vi "HolDrvCtrl_PackControllers.vi"(9 "thetaProfiledPID_CTRL":T1={"Controller"={"Kp"=0.0, "Ki"=0.0, "Kd"=0.0, "Period"=0.0, "Max_Integral"=1.0, "Min_Integral"=-1.0, "Max_Input"=0.0, "Min_Input"=0.0, "Continuous"=FALSE, "PositionError"=0.0, "VelocityError"=0.0, "PrevError"=0.0, "Total_Integral"=0.0, "PositionTolerance"=0.05, "VelocityTolerance"=9.99e+35, "SetPoint"=0.0, "Kf"=0.0, "Prev_Deriv"=0.0, "Prev_Deriv 2"=0.0, "DerivativeFilter"=FALSE, "Min_Output"=-9.99e+35, "Max_Output"=9.9e+35, "Prev_F_P"=0.0, "Prev_F_P_2"=0.0, "AntiWindupActive"=FALSE, "Measurement"=0.0, "IntegralZone"=9.9e+30}, "Goal"={"Position"=0.0, "Velocity"=0.0}, "Setpoint"={"Position"=0.0, "Velocity"=0.0}, "Constraint"={"MaxVelocity"=0.0, "MaxAcceleration"=0.0}} {"Constraint"."MaxAcceleration" format="%16_6e"; "Constraint"."MaxVelocity" format="%16_6e"; "Setpoint"."Velocity" format="%16_6e"; "Setpoint"."Position" format="%16_6e"; "Goal"."Velocity" format="%16_6e"; "Goal"."Position" format="%16_6e"; "Controller"."IntegralZone" format="%16_6e"; "Controller"."Measurement" format="%16_6e"; "Controller"."Prev_F_P_2" format="%16_6e"; "Controller"."Prev_F_P" format="%16_6e"; "Controller"."Max_Output" format="%16_6e"; "Controller"."Min_Output" format="%16_6e"; "Controller"."Prev_Deriv 2" format="%16_6e"; "Controller"."Prev_Deriv" format="%16_6e"; "Controller"."Kf" format="%16_6e"; "Controller"."SetPoint" format="%16_6e"; "Controller"."VelocityTolerance" format="%16_6e"; "Controller"."PositionTolerance" format="%16_6e"; "Controller"."Total_Integral" format="%16_6e"; "Controller"."PrevError" format="%16_6e"; "Controller"."VelocityError" format="%16_6e"; "Controller"."PositionError" format="%16_6e"; "Controller"."Min_Input" format="%16_6e"; "Controller"."Max_Input" format="%16_6e"; "Controller"."Min_Integral" format="%16_6e"; "Controller"."Max_Integral" format="%16_6e"; "Controller"."Period" format="%16_6e"; "Controller"."Kd" format="%16_6e"; "Controller"."Ki" format="%16_6e"; "Controller"."Kp" format="%16_6e"}, 10 "Y PID Tuning":T5={"Kp"=0.0, "Ki"=0.0, "Kd"=0.0, "MaximumIntegral"=9.9e+30, "MinimumIntegral"=-9.9e+30, "IntegralZone"=9.9e+30}, 11 "X PID Tuning":T5={"Kp"=0.0, "Ki"=0.0, "Kd"=0.0, "MaximumIntegral"=9.9e+30, "MinimumIntegral"=-9.9e+30, "IntegralZone"=9.9e+30}) -> (3 "HOLONOMIC_CTRL_PACK_TUNING":T6={"X PID Tuning"={"Kp"=0.0, "Ki"=0.0, "Kd"=0.0, "MaximumIntegral"=9.9e+30, "MinimumIntegral"=-9.9e+30, "IntegralZone"=9.9e+30}, "Y PID Tuning"={"Kp"=0.0, "Ki"=0.0, "Kd"=0.0, "MaximumIntegral"=9.9e+30, "MinimumIntegral"=-9.9e+30, "IntegralZone"=9.9e+30}, "thetaProfiledPID_CTRL"={"Controller"={"Kp"=0.0, "Ki"=0.0, "Kd"=0.0, "Period"=0.0, "Max_Integral"=1.0, "Min_Integral"=-1.0, "Max_Input"=0.0, "Min_Input"=0.0, "Continuous"=FALSE, "PositionError"=0.0, "VelocityError"=0.0, "PrevError"=0.0, "Total_Integral"=0.0, "PositionTolerance"=0.05, "VelocityTolerance"=9.99e+35, "SetPoint"=0.0, "Kf"=0.0, "Prev_Deriv"=0.0, "Prev_Deriv 2"=0.0, "DerivativeFilter"=FALSE, "Min_Output"=-9.99e+35, "Max_Output"=9.9e+35, "Prev_F_P"=0.0, "Prev_F_P_2"=0.0, "AntiWindupActive"=FALSE, "Measurement"=0.0, "IntegralZone"=9.9e+30}, "Goal"={"Position"=0.0, "Velocity"=0.0}, "Setpoint"={"Position"=0.0, "Velocity"=0.0}, "Constraint"={"MaxVelocity"=0.0, "MaxAcceleration"=0.0}}} {"thetaProfiledPID_CTRL"."Constraint"."MaxAcceleration" format="%16_6e"; "thetaProfiledPID_CTRL"."Constraint"."MaxVelocity" format="%16_6e"; "thetaProfiledPID_CTRL"."Setpoint"."Velocity" format="%16_6e"; "thetaProfiledPID_CTRL"."Setpoint"."Position" format="%16_6e"; "thetaProfiledPID_CTRL"."Goal"."Velocity" format="%16_6e"; "thetaProfiledPID_CTRL"."Goal"."Position" format="%16_6e"; "thetaProfiledPID_CTRL"."Controller"."IntegralZone" format="%16_6e"; "thetaProfiledPID_CTRL"."Controller"."Measurement" format="%16_6e"; "thetaProfiledPID_CTRL"."Controller"."Prev_F_P_2" format="%16_6e"; "thetaProfiledPID_CTRL"."Controller"."Prev_F_P" format="%16_6e"; "thetaProfiledPID_CTRL"."Controller"."Max_Output" format="%16_6e"; "thetaProfiledPID_CTRL"."Controller"."Min_Output" format="%16_6e"; "thetaProfiledPID_CTRL"."Controller"."Prev_Deriv 2" format="%16_6e"; "thetaProfiledPID_CTRL"."Controller"."Prev_Deriv" format="%16_6e"; "thetaProfiledPID_CTRL"."Controller"."Kf" format="%16_6e"; "thetaProfiledPID_CTRL"."Controller"."SetPoint" format="%16_6e"; "thetaProfiledPID_CTRL"."Controller"."VelocityTolerance" format="%16_6e"; "thetaProfiledPID_CTRL"."Controller"."PositionTolerance" format="%16_6e"; "thetaProfiledPID_CTRL"."Controller"."Total_Integral" format="%16_6e"; "thetaProfiledPID_CTRL"."Controller"."PrevError" format="%16_6e"; "thetaProfiledPID_CTRL"."Controller"."VelocityError" format="%16_6e"; "thetaProfiledPID_CTRL"."Controller"."PositionError" format="%16_6e"; "thetaProfiledPID_CTRL"."Controller"."Min_Input" format="%16_6e"; "thetaProfiledPID_CTRL"."Controller"."Max_Input" format="%16_6e"; "thetaProfiledPID_CTRL"."Controller"."Min_Integral" format="%16_6e"; "thetaProfiledPID_CTRL"."Controller"."Max_Integral" format="%16_6e"; "thetaProfiledPID_CTRL"."Controller"."Period" format="%16_6e"; "thetaProfiledPID_CTRL"."Controller"."Kd" format="%16_6e"; "thetaProfiledPID_CTRL"."Controller"."Ki" format="%16_6e"; "thetaProfiledPID_CTRL"."Controller"."Kp" format="%16_6e"})   [LabVIEW 2019, in "Trajectory_Library.lvlib"]
doc: "Pack controller tuning configuration for Holonomic Drive Controller.\n\n\nInputs:\n - X PID Tuning - Input from PACK PROF PID VI\n - Y PID Tuning - Input from PACK PROF PID VI\n - thetaController -- A profiled PID controller to respond to error in angle.\n\nOutputs:\n -- Holonomic_Ctrl_Packed -- cluster - packed controller configuration."
uses:
  Trajectory_Library.lvlib
  TypeDef/HOLONOMIC_PACK_TUNING.ctl
  TypeDef/PID_TUNING.ctl
  TypeDef/PROFILED_PID_CONTROLLER.ctl
  TypeDef/PID_CONTROLLER.ctl
  TypeDef/TRAPEZOID_PROFILE_STATE.ctl
  TypeDef/TRAPEZOID_PROFILE_CONSTRAINT.ctl
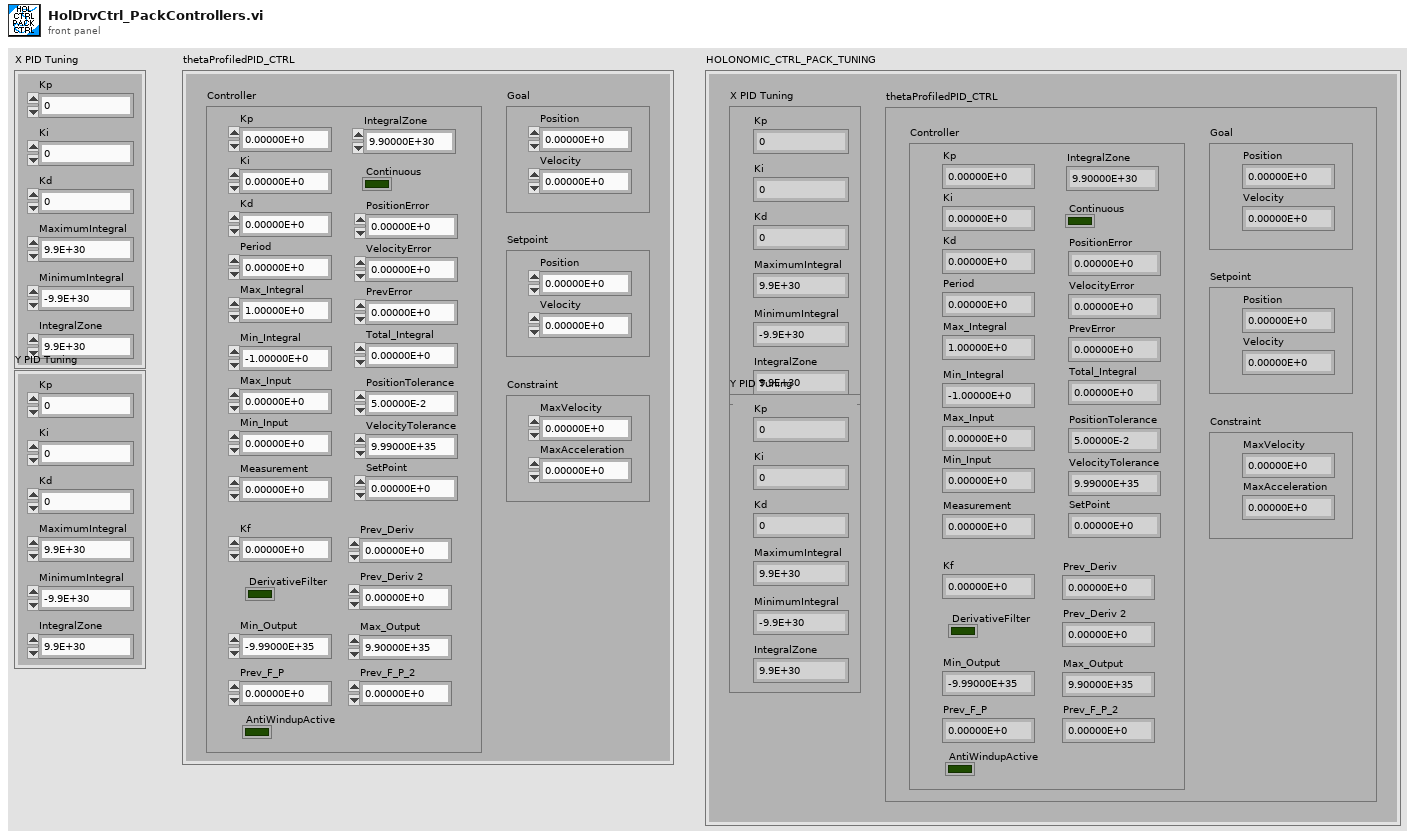
[diagram p1: front panel]
types:
  T1 = typedef "Trajectory_Library.lvlib/PROFILED_PID_CONTROLLER.ctl" = cluster{"Controller":T2, "Goal":T3, "Setpoint":T3, "Constraint":T4}
  T2 = typedef "Trajectory_Library.lvlib/PID_CONTROLLER.ctl" = cluster{"Kp":dbl, "Ki":dbl, "Kd":dbl, "Period":dbl, "Max_Integral":dbl, "Min_Integral":dbl, "Max_Input":dbl, "Min_Input":dbl, "Continuous":bool, "PositionError":dbl, "VelocityError":dbl, "PrevError":dbl, "Total_Integral":dbl, "PositionTolerance":dbl, "VelocityTolerance":dbl, "SetPoint":dbl, "Kf":dbl, "Prev_Deriv":dbl, "Prev_Deriv 2":dbl, "DerivativeFilter":bool, "Min_Output":dbl, "Max_Output":dbl, "Prev_F_P":dbl, "Prev_F_P_2":dbl, "AntiWindupActive":bool, "Measurement":dbl, "IntegralZone":dbl}
  T3 = typedef "Trajectory_Library.lvlib/TRAPEZOID_PROFILE_STATE.ctl" = cluster{"Position":dbl, "Velocity":dbl}
  T4 = typedef "Trajectory_Library.lvlib/TRAPEZOID_PROFILE_CONSTRAINT.ctl" = cluster{"MaxVelocity":dbl, "MaxAcceleration":dbl}
  T5 = typedef "Trajectory_Library.lvlib/PID_TUNING.ctl" = cluster{"Kp":dbl, "Ki":dbl, "Kd":dbl, "MaximumIntegral":dbl, "MinimumIntegral":dbl, "IntegralZone":dbl}
  T6 = typedef "Trajectory_Library.lvlib/HOLONOMIC_PACK_TUNING.ctl" = cluster{"X PID Tuning":T5, "Y PID Tuning":T5, "thetaProfiledPID_CTRL":T1}
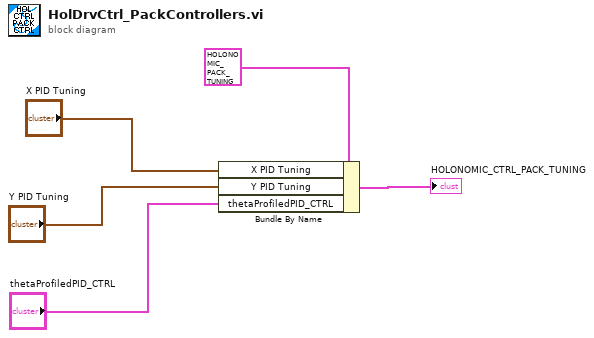
[diagram p0: block diagram]
diagram:
  n1 = Bundle By Name(cluster=T6 {"X PID Tuning"={"Kp"=0.0, "Ki"=0.0, "Kd"=0.0, "MaximumIntegral"=9.9e+30, "MinimumIntegral"=-9.9e+30, "IntegralZone"=9.9e+30}, "Y PID Tuning"={"Kp"=0.0, "Ki"=0.0, "Kd"=0.0, "MaximumIntegral"=9.9e+30, "MinimumIntegral"=-9.9e+30, "IntegralZone"=9.9e+30}, "thetaProfiledPID_CTRL"={"Controller"={"Kp"=0.0, "Ki"=0.0, "Kd"=0.0, "Period"=0.0, "Max_Integral"=1.0, "Min_Integral"=-1.0, "Max_Input"=0.0, "Min_Input"=0.0, "Continuous"=FALSE, "PositionError"=0.0, "VelocityError"=0.0, "PrevError"=0.0, "Total_Integral"=0.0, "PositionTolerance"=0.05, "VelocityTolerance"=9.99e+35, "SetPoint"=0.0, "Kf"=0.0, "Prev_Deriv"=0.0, "Prev_Deriv 2"=0.0, "DerivativeFilter"=FALSE, "Min_Output"=-9.99e+35, "Max_Output"=9.9e+35, "Prev_F_P"=0.0, "Prev_F_P_2"=0.0, "AntiWindupActive"=FALSE, "Measurement"=0.0, "IntegralZone"=9.9e+30}, "Goal"={"Position"=0.0, "Velocity"=0.0}, "Setpoint"={"Position"=0.0, "Velocity"=0.0}, "Constraint"={"MaxVelocity"=0.0, "MaxAcceleration"=0.0}}} ("HOLONOMIC_CTRL_PACK_TUNING"), "X PID Tuning"="X PID Tuning", "Y PID Tuning"="Y PID Tuning", "thetaProfiledPID_CTRL"="thetaProfiledPID_CTRL") -> (→"HOLONOMIC_CTRL_PACK_TUNING":T6)
